vi "DataParser.vi"(10 "Control":enum16{"Init", "ParseNewData"}(ring), 11 "NewData":u8[](array[numeric])) -> ()   [LabVIEW 2017]
uses:
  SimpleFrameParserState.ctl
panel:
  out "SimpleFrameParserStateOut":T1
  out "Position":i16[](array[numeric])
  out "CurrentC":i16[](array[numeric])
  out "CurrentB":i16[](array[numeric])
  out "CurrentA":i16[](array[numeric])
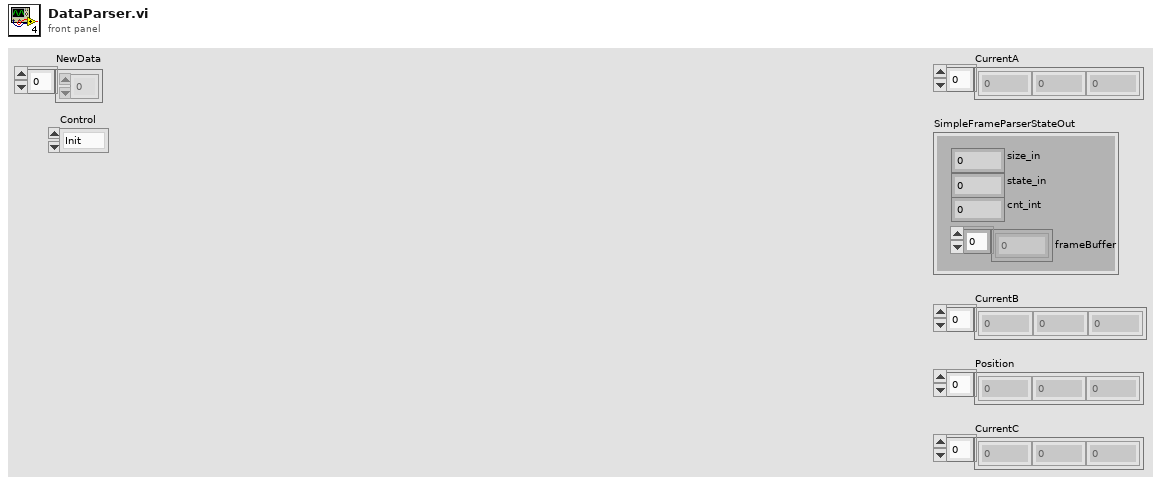
[diagram p1: front panel]
types:
  T1 = typedef "SimpleFrameParserState.ctl" = cluster{"state_in":i32, "cnt_int":i32, "size_in":i32, "frameBuffer":u8[]}
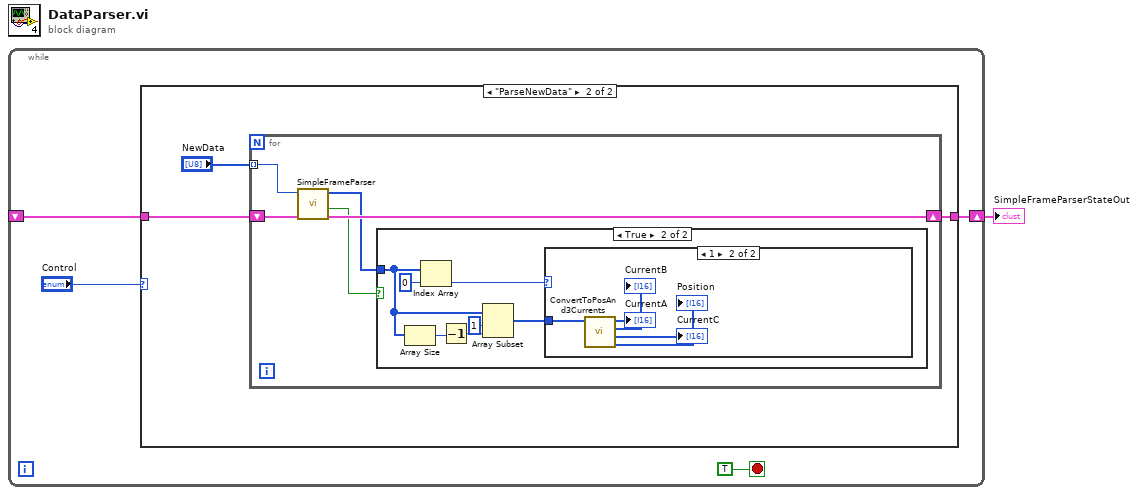
[diagram p0: block diagram]
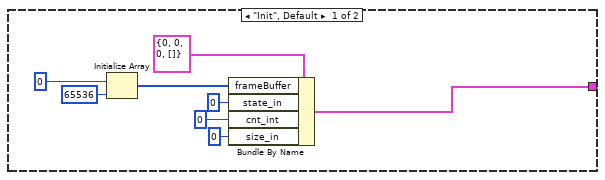
[diagram p2: hidden frame]
diagram:
  n1 = while {
    shift-right: [w4] -> w1
    shift-left: _ -> [w3]
    stop <- TRUE stop-if-true
    n2 = case shown="\"ParseNewData\"" "Control" {
      tunnel: [w10 w14] -> w4
      tunnel: w3 -> [_ w15]
      frame "Init", Default {
        n3 = Initialize Array(u8 0 ("input variable"), 65536 ("dimension size")) -> (w9:u8[])
        n4 = Bundle By Name(cluster=T1 {"state_in"=0, "cnt_int"=0, "size_in"=0, "frameBuffer"=[]} ("SimpleFrameParserState"), "frameBuffer"=w9, "state_in"=0, "cnt_int"=0, "size_in"=0) -> (w10:T1)
      }
      frame "ParseNewData" {
        n5 = for {
          tunnel: "NewData" -> [w20] mode=indexing
          shift-right: [w19] -> w14
          shift-left: w15 -> [w21]
          n6 = call "SimpleFrameParser.vi"("SimpleFrameParserState"=w21, "data"=w20) -> ("SimpleFrameParserStateOut"=w19:T1, "frameComplete"=w18:bool, "frame_data"=w17:u8[])  [unwired: 5 in]
          n7 = case shown="True" w18 {
            tunnel: w17 -> [_ w24]
            frame False {
            }
            frame True {
              n8 = Array Size(array=w24) -> (size(s)=w27:i32)
              n9 = Index Array(array=w24, index=0) -> (element=w23:u8)
              n10 = Decrement(x=w27) -> (x-1=w26:i32)
              n11 = Array Subset(array=w24, index=1, length=w26) -> (w22:u8[])
              n12 = case shown="1" w23 {
                tunnel: w22 -> [_ w33]
                frame 0, Default {
                }
                frame 1 {
                  n13 = call "ConvertToPosAnd3Currents.vi"("dataFrame"=w33) -> ("Position"=→"Position":i16[], "CurrentC"=→"CurrentC":i16[], "CurrentB"=→"CurrentB":i16[], "CurrentA"=→"CurrentA":i16[])  [unwired: 7 in]
                }
              }
            }
          }
        }
      }
    }
  }
  "SimpleFrameParserStateOut" <- w1
